vi "选择补传参数对话框.vi"() -> (3 "参数数值out":T1={"CODMn"=TRUE, "CODCr"=TRUE, "DO"=TRUE, "铜"=TRUE, "PH"=TRUE, "氨氮"=TRUE, "比电导率"=TRUE, "水温"=TRUE, "COD"=TRUE, "浊度"=TRUE, "总氮"=TRUE, "总磷"=TRUE, "叶绿素a"=TRUE, "藻密度"=TRUE, "水位"=TRUE, "流速"=TRUE, "瞬时流量"=TRUE, "累积流量"=TRUE, "亚硝氮"=TRUE, "硫化物"=TRUE, "ORP"=TRUE, "铅"=TRUE, "镉"=TRUE, "锌"=TRUE, "镍"=TRUE, "锰"=TRUE, "汞"=TRUE, "气温"=TRUE, "气压"=TRUE, "风速"=TRUE, "风向"=TRUE, "盐度"=TRUE, "磷酸盐"=TRUE, "硝氮"=TRUE, "氟化物"=TRUE, "挥发酚"=TRUE, "氯化物"=TRUE})   [LabVIEW 2016, in "数据传输系统-02.lvlib"]
uses:
  <vilib>/Utility/miscctls.llb/LVPointTypeDef.ctl
panel:
  in  "取消全选":bool
  in  "取消":bool
  in  "确定":bool
  in  "全选":bool
  in  "参数数值":T1={"CODMn"=TRUE, "CODCr"=TRUE, "DO"=TRUE, "铜"=TRUE, "PH"=TRUE, "氨氮"=TRUE, "比电导率"=TRUE, "水温"=TRUE, "COD"=TRUE, "浊度"=TRUE, "总氮"=TRUE, "总磷"=TRUE, "叶绿素a"=TRUE, "藻密度"=TRUE, "水位"=TRUE, "流速"=TRUE, "瞬时流量"=TRUE, "累积流量"=TRUE, "亚硝氮"=TRUE, "硫化物"=TRUE, "ORP"=TRUE, "铅"=TRUE, "镉"=TRUE, "锌"=TRUE, "镍"=TRUE, "锰"=TRUE, "汞"=TRUE, "气温"=TRUE, "气压"=TRUE, "风速"=TRUE, "风向"=TRUE, "盐度"=TRUE, "磷酸盐"=TRUE, "硝氮"=TRUE, "氟化物"=TRUE, "挥发酚"=TRUE, "氯化物"=TRUE}
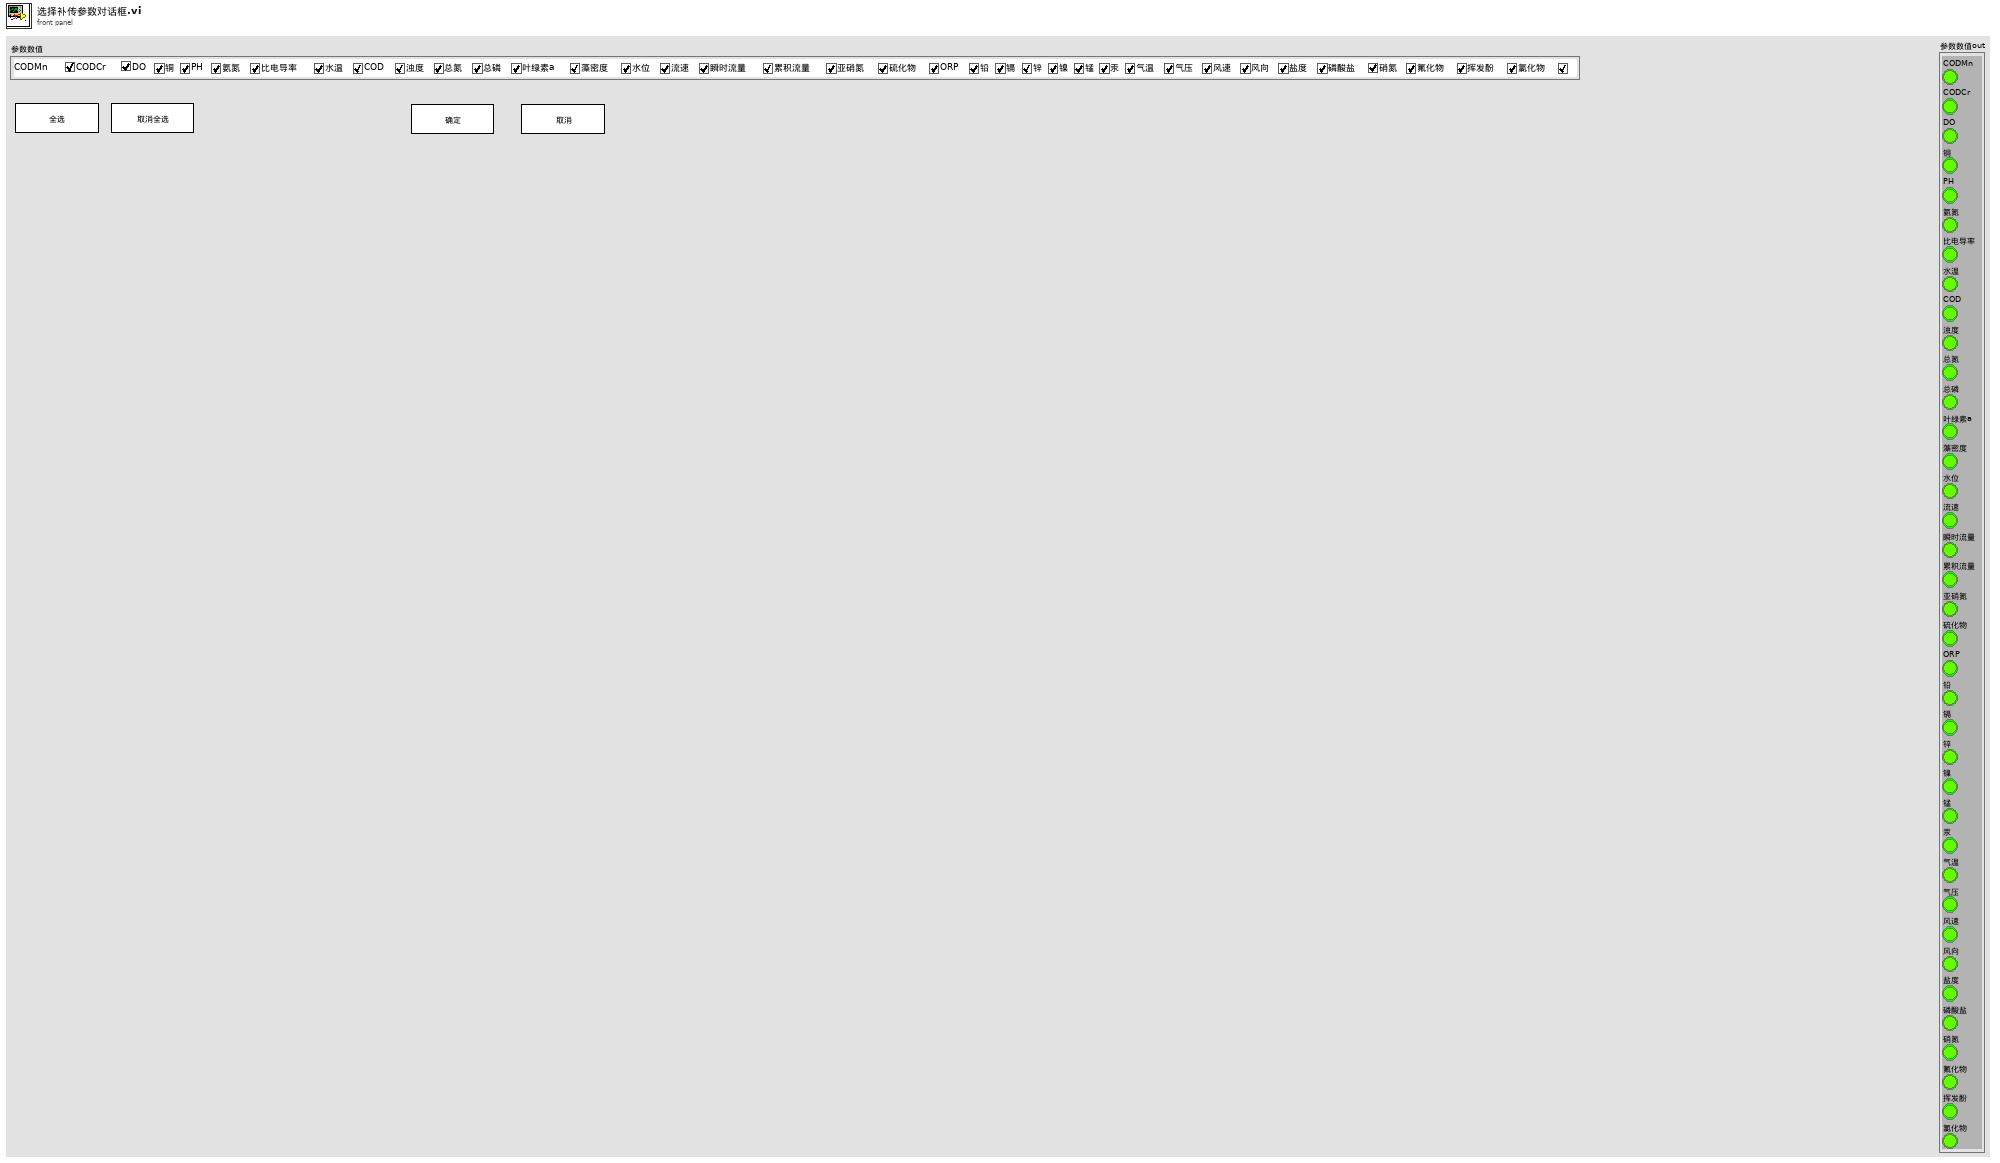
[diagram p1: front panel]
types:
  T1 = cluster{"CODMn":bool, "CODCr":bool, "DO":bool, "铜":bool, "PH":bool, "氨氮":bool, "比电导率":bool, "水温":bool, "COD":bool, "浊度":bool, "总氮":bool, "总磷":bool, "叶绿素a":bool, "藻密度":bool, "水位":bool, "流速":bool, "瞬时流量":bool, "累积流量":bool, "亚硝氮":bool, "硫化物":bool, "ORP":bool, "铅":bool, "镉":bool, "锌":bool, "镍":bool, "锰":bool, "汞":bool, "气温":bool, "气压":bool, "风速":bool, "风向":bool, "盐度":bool, "磷酸盐":bool, "硝氮":bool, "氟化物":bool, "挥发酚":bool, "氯化物":bool}
  T2 = typedef "LVPointTypeDef.ctl" = cluster{"Horizontal":i16, "Vertical":i16}
  T3 = cluster{"[0]":bool, "[1]":bool, "[2]":bool, "[3]":bool, "[4]":bool, "[5]":bool, "[6]":bool, "[7]":bool, "[8]":bool, "[9]":bool, "[10]":bool, "[11]":bool, "[12]":bool, "[13]":bool, "[14]":bool, "[15]":bool, "[16]":bool, "[17]":bool, "[18]":bool, "[19]":bool, "[20]":bool, "[21]":bool, "[22]":bool, "[23]":bool, "[24]":bool, "[25]":bool, "[26]":bool, "[27]":bool, "[28]":bool, "[29]":bool, "[30]":bool, "[31]":bool, "[32]":bool, "[33]":bool, "[34]":bool, "[35]":bool, "[36]":bool}
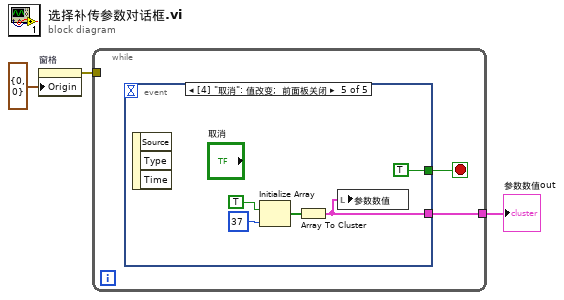
[diagram p0: block diagram]
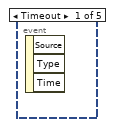
[diagram p2: hidden frame]
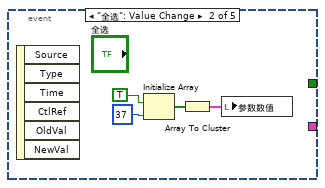
[diagram p3: hidden frame]
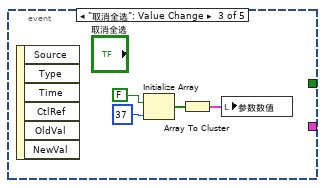
[diagram p4: hidden frame]
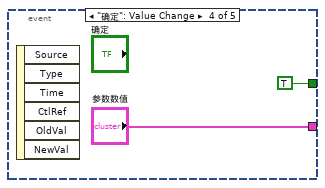
[diagram p5: hidden frame]
diagram:
  n1 = property on="窗格" class="Pane"("Origin"=T2 {"Horizontal"=0, "Vertical"=0} ("原点")) -> (error out=w1:errorcluster)  [unwired: 2 in, 1 out]
  n2 = while {
    tunnel: [w4] -> w3
    tunnel: w1 -> [_]
    stop <- w5 stop-if-true
    n3 = event shown="[4] \"取消\": 值改变;  前面板关闭" {
      selector: _ -> [_ _ _ _ _]
      dyn-events: _ -> [_ _ _ _ _]
      timeout: _ -> [_ _ _ _ _]
      tunnel: [_ _ _ TRUE TRUE] -> w5
      tunnel: [_ _ _ "参数数值" w16] -> w4
      event Timeout {
        n4 = event-data() -> ()  [unwired: 1 in, 3 out]
      }
      event "全选": Value Change {
        n5 = event-data() -> ()  [unwired: 1 in, 6 out]
        n6 = Initialize Array(TRUE, 37 ("维数大小")) -> (w8:bool[])
        n7 = Array To Cluster(array=w8) -> (cluster=w6:T3)
        n8 = local write "参数数值"(w6) -> ()
      }
      event "取消全选": Value Change {
        n9 = event-data() -> ()  [unwired: 1 in, 6 out]
        n10 = Initialize Array(FALSE, 37 ("维数大小")) -> (w12:bool[])
        n11 = Array To Cluster(array=w12) -> (cluster=w10:T3)
        n12 = local write "参数数值"(w10) -> ()
      }
      event "确定": Value Change {
        n13 = event-data() -> ()  [unwired: 1 in, 6 out]
      }
      event "取消": Value Change; Panel Close {
        n14 = event-data() -> ()  [unwired: 1 in, 3 out]
        n15 = Initialize Array(TRUE, 37 ("维数大小")) -> (w18:bool[])
        n16 = Array To Cluster(array=w18) -> (cluster=w16:T3)
        n17 = local write "参数数值"(w16) -> ()
      }
    }
  }
  "参数数值out" <- w3
